vi "Ratio2pH.vi"(1 "SNARF":T1, 2 "Smoothed Array":dbl[](array[numeric])) -> (0 "Smoothed Array 2":dbl[](array[numeric]))   [LabVIEW 2010]
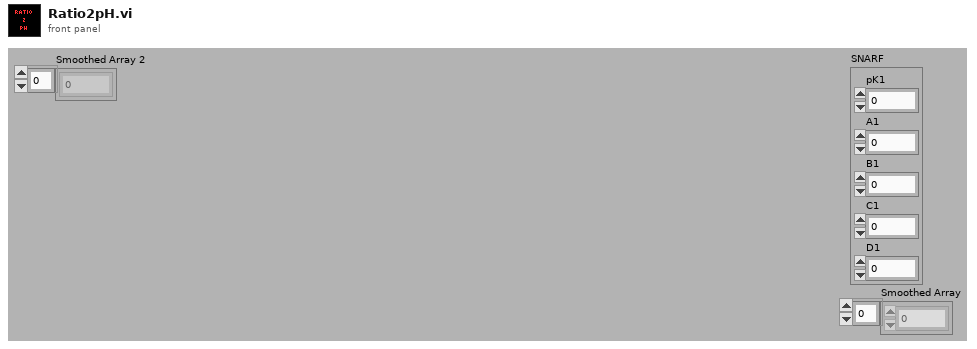
[diagram p1: front panel]
types:
  T1 = cluster{"pK1":dbl, "A1":dbl, "B1":dbl, "C1":dbl, "D1":dbl}
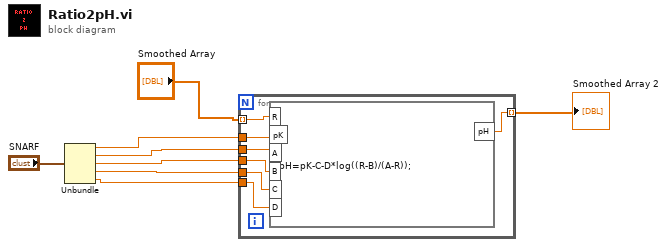
[diagram p0: block diagram]
diagram:
  n1 = Unbundle("SNARF") -> ("pK1"=w7:dbl, "A1"=w6:dbl, "B1"=w5:dbl, "C1"=w4:dbl, "D1"=w3:dbl)
  n2 = for {
    tunnel: w6 -> [w14]
    tunnel: w5 -> [w13]
    tunnel: w4 -> [w12]
    tunnel: w3 -> [w11]
    tunnel: w7 -> [w15]
    tunnel: "Smoothed Array" -> [w10] mode=indexing
    tunnel: [w9] -> w1 mode=indexing
    n3 = formula code="pH=pK-C-D*log((R-B)/(A-R));"("R"=w10, "pK"=w15, "A"=w14, "B"=w13, "C"=w12, "D"=w11) -> ("pH"=w9:dbl)
  }
  "Smoothed Array 2" <- w1
